vi "Is_any_motor_moving.vi"(8 "error in (no error)":errorcluster, 11 "VISA resource name":refnum<visa-resource-name>) -> (0 "error out":errorcluster={"status"=FALSE, "code"=1073676294, "source"="VISA Read in write_read.vi"}, 1 "Motor Moving (M1/2/3/4)":bool[](array[boolean]), 2 "Motor Moving":bool, 3 "VISA ressource out":refnum<visa-resource-name>)   [LabVIEW 2018]
uses:
  MCode_LV_86/Set Parameter.ctl
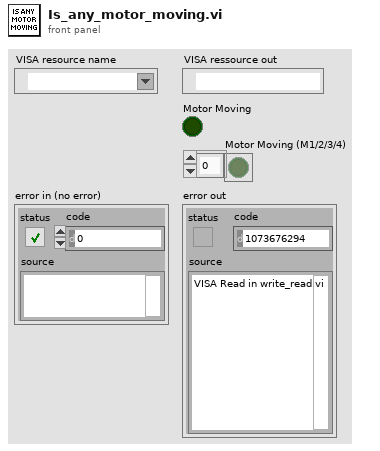
[diagram p1: front panel]
types:
  T1 = typedef "Set Parameter.ctl" = enum16{"Acceleration (A)", "Baud Rate (BD)", "Counter 1 (C1)", "Counter 2 (C2)", "Control C Software Reset (CE)", "Check Sum Enable (CK)", "Clock Mode (CM)", "Clock Mode Ratio (CR)", "Clock Mode Out Step Width (CW)", "Deceleration (D)", "Digital Filtering, Input 1 (D1)", "Digital Filtering, Input 2 (D2)", "Digital Filtering, Input 3 (D3)", "Digital Filtering, Input 4 (D4)", "Digital Filtering, Input 5 (D5)", "Digital Filtering, Input 9 (D9)", "Digital Filtering, Input 10 (D10)", "Digital Filtering, Input 11 (D11)", "Digital Filtering, Input 12 (D12)", "Deadband (DB)", "Decrement Variable (DC)", "Enable/Disable Drive (DE)", "Device Name (DN)", "End Program Execution (E)", "Encoder Function Enable (EE)", "Error Flag (EF)", "Encoder Lines (EL)", "Echo Mode (EM)", "Error Value (ER)", "Escape (ES)", "Execute Program at Address (EX)", "Firmware Version (VR)", "Hold (H)", "Hold Current (HC)", "Hold Current Delay Time (HI)", "Home to Encoder Index (HM)", "Home to Home Switch (HT)", "Increment Variable (IC)", "Initialize Parameters to NVM (IP)", "Input into Variable (IV)", "Jog Enable (JE)", "Limit Stop Mode (LM)", "Move Absolute (MA)", "Move Relative (MR)", "MicroStepping Select (MS)", "Motor Settling Delay Time (MT)", "Moving [Flag] (MV)", "Output 1 (O1)", "Output 2 (O2)", "Output 3 (O3)", "Output 4 (O4)", "Output 9 (O9)", "Output 10 (O10)", "Output 11 (O11)", "Output 12 (O12)", "Output High Byte (9-12) (OH)", "Output Low Byte (1-4) (OL)", "Output Total (1-4 and 9-12) (OT)", "Position (P)", "Position Maintenance (PM)", "Party Mode (PY)", "Register 1 (R1)", "Register 2 (R2)", "Register 3 (R3)", "Register 4 (R4)", "Reset Error(\\03)", "Run Current (RC)", "Stall Factor (SF)", "Slew (SL)", "Stall Mode Set (SM)", "Upgrade Firmware (UG)", "Velocity Initial (VI)", "Velocity Maximum (VM)", "Current1 (I1)", "Current2 (I2)", "Current3 (I3)", "Current4 (I4)", "Current5 (I5)", "Current6 (I6)", "Save (S)"}
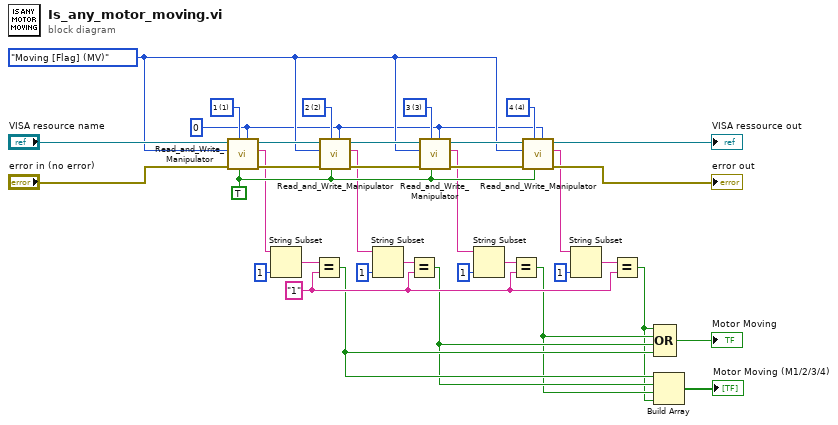
[diagram p0: block diagram]
diagram:
  w19 = u32 0 ("additional waiting time (0)")
  w21 = "1" ("y")
  w23 = u16 4 items=["none", "1", "2", "3", "4", "all"] ("Motor")
  w24 = u16 3 items=["none", "1", "2", "3", "4", "all"] ("Motor")
  w25 = u16 2 items=["none", "1", "2", "3", "4", "all"] ("Motor")
  w36 = u16 1 items=["none", "1", "2", "3", "4", "all"] ("Motor")
  w32 = TRUE ("Print?")
  w22 = Set_Parameter."Moving [Flag] (MV)" ("Command")
  n1 = call "Read_and_Write_Manipulator.vi"("additional waiting time (0)"=w19, "Print?"=w32, "Motor"=w36, "error in (no error)"="error in (no error)", "Command"=w22, "VISA resource name"="VISA resource name") -> ("error out"=w31:errorcluster, "Answer"=w16:string, "VISA ressource out"=w35:refnum<visa-resource-name>)  [unwired: 1 in, 2 out]
  n2 = String Subset(string=w16, length (rest)=1 ("length (rest)")) -> (substring=w15:string)  [unwired: 1 in]
  n3 = Equal?(x=w15, y=w21) -> (x = y?=w6:bool)
  n4 = call "Read_and_Write_Manipulator.vi"("additional waiting time (0)"=w19, "Print?"=w32, "Motor"=w25, "error in (no error)"=w31, "Command"=w22, "VISA resource name"=w35) -> ("error out"=w30:errorcluster, "Answer"=w13:string, "VISA ressource out"=w34:refnum<visa-resource-name>)  [unwired: 1 in, 2 out]
  n5 = String Subset(string=w13, length (rest)=1 ("length (rest)")) -> (substring=w12:string)  [unwired: 1 in]
  n6 = Equal?(x=w12, y=w21) -> (x = y?=w5:bool)
  n7 = call "Read_and_Write_Manipulator.vi"("additional waiting time (0)"=w19, "Print?"=w32, "Motor"=w24, "error in (no error)"=w30, "Command"=w22, "VISA resource name"=w34) -> ("error out"=w29:errorcluster, "Answer"=w10:string, "VISA ressource out"=w33:refnum<visa-resource-name>)  [unwired: 1 in, 2 out]
  n8 = String Subset(string=w10, length (rest)=1 ("length (rest)")) -> (substring=w9:string)  [unwired: 1 in]
  n9 = Equal?(x=w9, y=w21) -> (x = y?=w4:bool)
  n10 = call "Read_and_Write_Manipulator.vi"("additional waiting time (0)"=w19, "Print?"=w32, "Motor"=w23, "error in (no error)"=w29, "Command"=w22, "VISA resource name"=w33) -> ("error out"=→"error out":errorcluster, "Answer"=w8:string, "VISA ressource out"=→"VISA ressource out":refnum<visa-resource-name>)  [unwired: 1 in, 2 out]
  n11 = String Subset(string=w8, length (rest)=1 ("length (rest)")) -> (substring=w7:string)  [unwired: 1 in]
  n12 = Equal?(x=w7, y=w21) -> (x = y?=w3:bool)
  n13 = Compound Arithmetic op=OR(w3, w4, w5, w6) -> (→"Motor Moving":bool)
  n14 = Build Array(w6, w5, w4, w3) -> (→"Motor Moving (M1/2/3/4)":bool[])
